vi "Launch Listener.vi"(11 "Log Sinks in":refnum<class "Log Sinks.lvclass">) -> (0 "error out":errorcluster, 3 "Log Sinks out":refnum<class "Log Sinks.lvclass">)   [LabVIEW 2019, in "TSC Event Logger.lvlib" / "Log Sinks.lvclass"]
uses:
  Log Sinks.lvclass
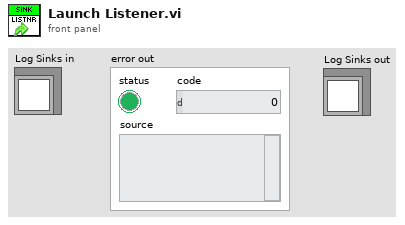
[diagram p1: front panel]
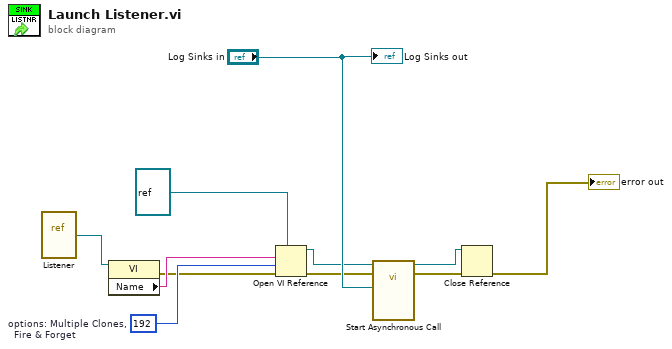
[diagram p0: block diagram]
diagram:
  w6 = 192  # options: Multiple Clones,   Fire & Forget
  n1 = vi-ref "Listener.vi"() -> (w3:refnum<vi>)
  n2 = property class="VI"(reference=w3) -> (error out=w2:errorcluster, "Name"=w5:string)  [unwired: 1 in, 1 out]
  n3 = Open VI Reference(type specifier VI Refnum (for type only)=refnum<vi> refnum, vi path=w5, options=w6, error in (no error)=w2) -> (vi reference=w8:refnum<vi>, error out=w4:errorcluster)  [unwired: 2 in]
  n4 = call-by-ref "Start Asynchronous Call"(reference=w8, error in=w4, "Log Sinks"="Log Sinks in") -> (reference out=w10:refnum<vi>, error out=w9:errorcluster)  [unwired: 11 in]
  n5 = Close Reference(reference=w10, error in (no error)=w9) -> (error out=→"error out":errorcluster)
  "Log Sinks out" <- "Log Sinks in"
